vi "Close.vi"(8 "error in":errorcluster, 11 "Current Limits in":refnum<class "Current Limits.lvclass">) -> (0 "error out":errorcluster, 3 "Current Limits out":refnum<class "Current Limits.lvclass">)   [LabVIEW 2023, in "Current Limits.lvclass"]
uses:
  Current Limits.lvclass
  Current Limits.lvclass/Current Limits.ctl
  <vilib>/ADAS Replay HIL/AdasHilServices/AdasHilServices Fill In Error Info Ex.vi
  <vilib>/ADAS Replay HIL/AdasHilServices/AdasHilChannelServices.lvlib
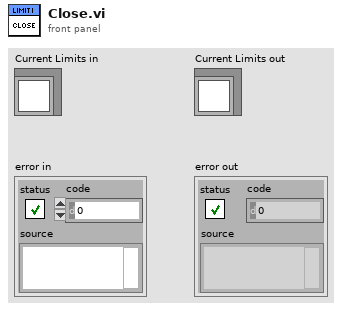
[diagram p1: front panel]
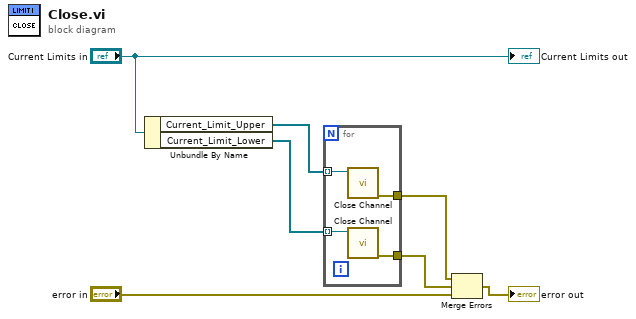
[diagram p0: block diagram]
diagram:
  n1 = Unbundle By Name("Current Limits in") -> ("Current_Limit_Upper"=w6:refnum<k21>[], "Current_Limit_Lower"=w5:refnum<k21>[])
  n2 = for {
    tunnel: w6 -> [w11] mode=indexing
    tunnel: w5 -> [w10] mode=indexing
    tunnel: [w9] -> w2
    tunnel: [w8] -> w1
    n3 = call <vilib>:"Close Channel.vi"("ADAS HIL Channel"=w11) -> ("error out"=w8:errorcluster)  [unwired: 10 in]
    n4 = call <vilib>:"Close Channel.vi"("ADAS HIL Channel"=w10) -> ("error out"=w9:errorcluster)  [unwired: 10 in]
  }
  n5 = Merge Errors(w1, w2, "error in") -> (→"error out":errorcluster)
  "Current Limits out" <- "Current Limits in"
